vi "Fetch.vi"(8 "error in (no error)":errorcluster, 10 "maximum time (5s)":dbl[unit]=5000.0 caption="maximum time (5000 ms)", 11 "CS++DMM in":refnum<class "CS++DMM.lvclass">) -> (0 "error out":errorcluster, 2 "reading":dbl format="%^.2e", 3 "CS++DMM out":refnum<class "CS++DMM.lvclass">)   [LabVIEW 2013, in "CS++DMM.lvlib" / "CS++DMM.lvclass"]
doc: "This VI returns the value from a previously initiated measurement.\n\nYou must first call the IviDmm Initiate VI to initiate a measurement before calling this VI.\n\nNotes:\n\n(1) After this VI executes, the Reading parameter contains an actual reading or a value indicating that an over-range condition occurred.\n\n(2) If an over-range condition occurs, the Reading parameter contains an IEEE defined NaN (Not a Number) value and the VI returns the IVIDMM_WARN_OVER_RANGE (0x3FFA2001) warning code. \n\n(3) You can test the measurement value for an over-range conditiion by calling the IviDmm Is Over-Range VI.\n\n(4) The class driver returns a simulated measurement when this VI is called and the IviDmm>>Inherent IVI Settings>>User Options>>Simulate property is set to TRUE and the IviDmm>>Inherent IVI Settings>>User Options>>Use Specific Simulation property is set to FALSE. For information on how to configure a simulated measurement, refer to the online help manual.\n\n(5) This VI does not check the instrument status. Typically, you call this VI only in a sequence of calls to other low-level driver VIs. The sequence performs one operation. You use the low-level VIs to optimize one or more aspects of interaction with the instrument. If you want to check the instrument status, call the IviDmm Error-Query VI at the conclusion of the sequence."
uses:
  CS++DMM.lvclass
  CS++DMM.lvclass/CS++DMM.ctl
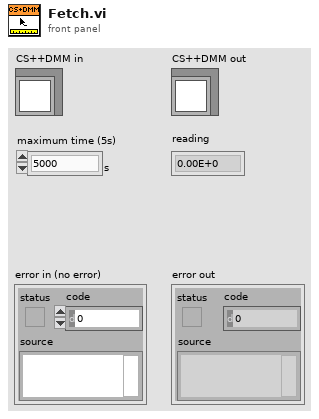
[diagram p1: front panel]
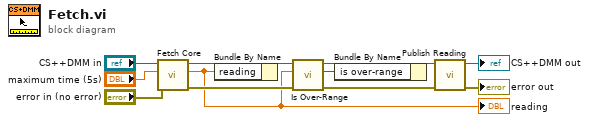
[diagram p0: block diagram]
diagram:
  n1 = call-dynamic "Fetch Core.vi"("error in (no error)"="error in (no error)", "maximum time (5s)"="maximum time (5s)", "CS++DMM in"="CS++DMM in") -> ("error out"=w7:errorcluster, "reading"=w2:dbl, "CS++DMM out"=w6:refnum<class "CS++DMM.lvclass">)  [unwired: 6 in]
  "reading" <- w2
  n2 = Bundle By Name(cluster=w6, "reading"=w2) -> (w3:refnum<class "CS++DMM.lvclass">)
  n3 = call-dynamic "Is Over-Range.vi"("measurement value"=w2, "CS++DMM in"=w3) -> ("is over-range"=w5:bool, "CS++DMM out"=w4:refnum<class "CS++DMM.lvclass">)  [unwired: 7 in, 1 out]
  n4 = Bundle By Name(cluster=w4, "is over-range"=w5) -> (w1:refnum<class "CS++DMM.lvclass">)
  n5 = call "Publish Reading.vi"("error in (no error)"=w7, "CS++DMM in"=w1) -> ("error out"=→"error out":errorcluster, "CS++DMM out"=→"CS++DMM out":refnum<class "CS++DMM.lvclass">)  [unwired: 8 in]
